vi "Resize Front Panel Main.vi"(0 "Left Listbox":refnum<vi>, 1 "Top Level VI":refnum<vi>, 2 "Stop":refnum<vi>, 3 "Number of Columns":i32=4, 7 "Left Splitter":refnum<vi>, 11 "error in (no error)":errorcluster, 12 "Left Pane Items":refnum<vi>[](array[refnum]), 13 "Mid Pane Items":refnum<vi>[](array[refnum])) -> (15 "error out":errorcluster)   [LabVIEW 2020]
uses:
  <vilib>/Utility/miscctls.llb/LVRectTypeDef.ctl
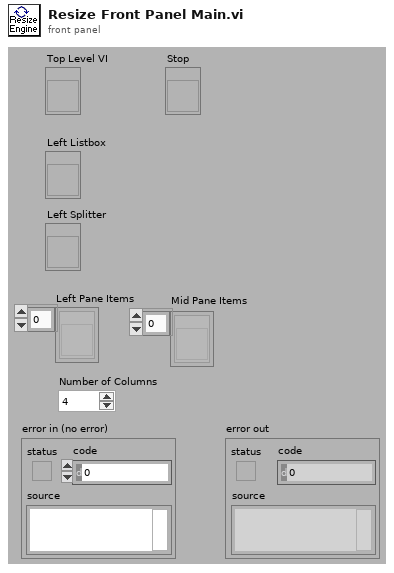
[diagram p1: front panel]
types:
  T1 = typedef "LVRectTypeDef.ctl" = cluster{"Left":i16, "Top":i16, "Right":i16, "Bottom":i16}
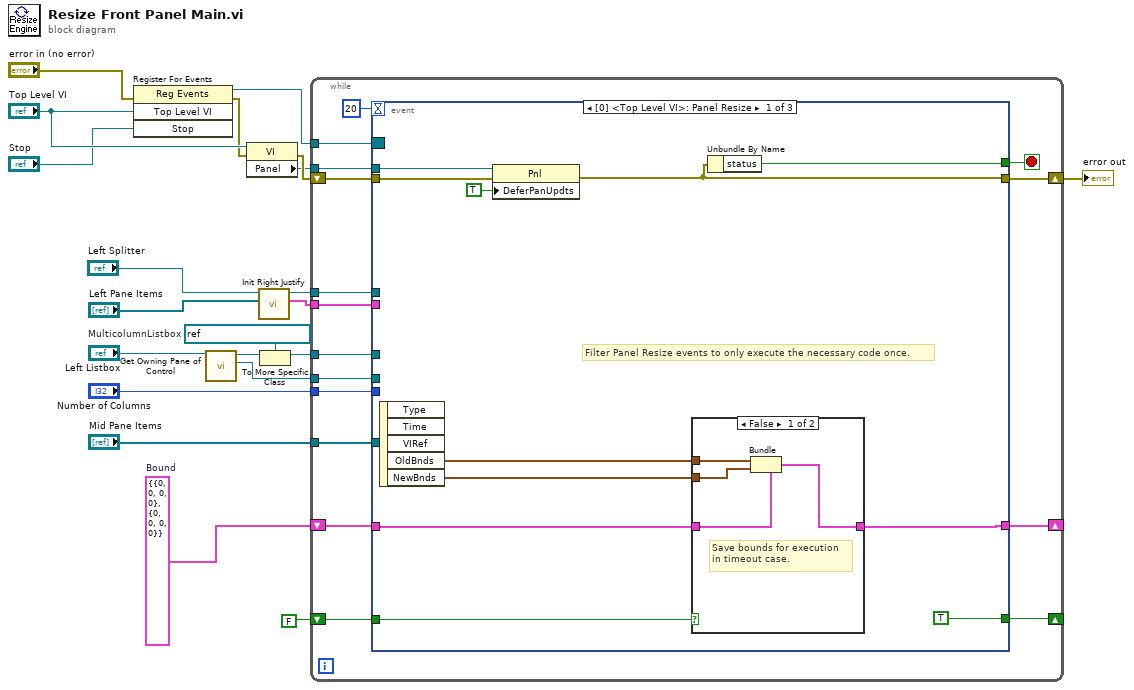
[diagram p0: block diagram]
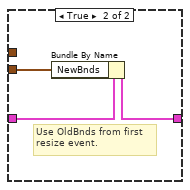
[diagram p2: hidden frame]
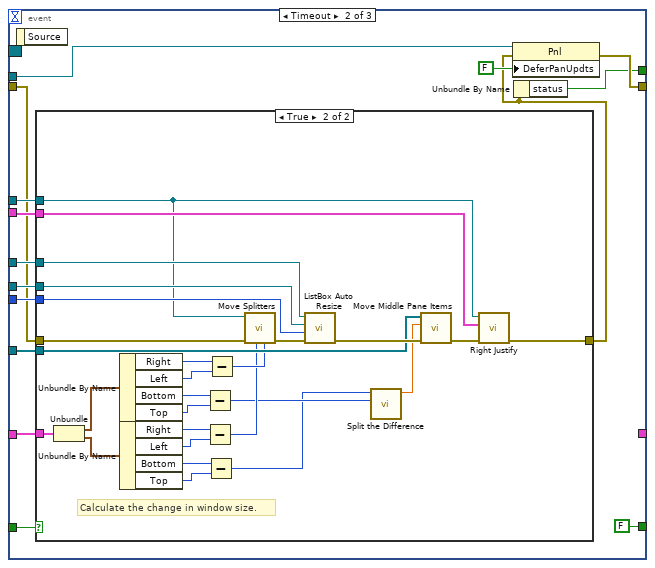
[diagram p3: hidden frame]
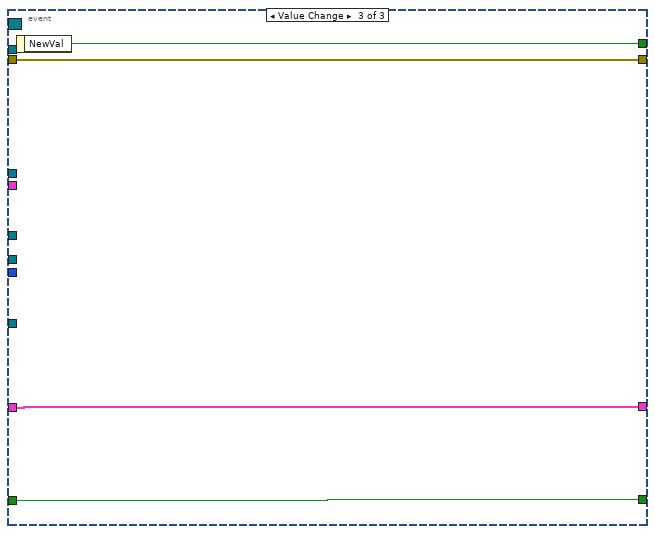
[diagram p5: hidden frame]
diagram:
  w2 = cluster{"OldBnds":T1, "NewBnds":T1} {"OldBnds"={"Left"=0, "Top"=0, "Right"=0, "Bottom"=0}, "NewBnds"={"Left"=0, "Top"=0, "Right"=0, "Bottom"=0}}  # Bound
  w4 = refnum<vi> refnum  # MulticolumnListbox
  n1 = register-events(error in="error in (no error)", "Top Level VI", "Stop") -> (reference out=w15:refnum<event-registration>, error out=w14:errorcluster)  [unwired: 1 in]
  n2 = call "Get Owning Pane of Control.vi"("Ctl Refnum"="Left Listbox") -> ("Owning Pane"=w7:refnum<vi>, "dup Ctl Refnum"=w6:refnum<vi>)  [unwired: 8 in, 1 out]
  n3 = property class="VI"(reference="Top Level VI", error in=w14) -> (error out=w13:errorcluster, "Panel"=w3:refnum<vi>)  [unwired: 1 out]
  n4 = call "Init Right Justify.vi"("Right Justified Items"="Left Pane Items", "Splitter Reference"="Left Splitter") -> ("Position Coordinates"=w18:cluster{refnum<vi>, i32}[], "Splitter Reference"=w20:refnum<vi>)  [unwired: 7 in, 1 out]
  n5 = To More Specific Class(target class=w4, reference=w6) -> (specific class reference=w5:refnum<vi>)  [unwired: 1 in, 1 out]
  n6 = while {
    tunnel: w3 -> [w36]
    tunnel: w18 -> [w34]
    tunnel: w20 -> [w33]
    tunnel: w15 -> [w32]
    tunnel: w5 -> [w31]
    shift-right: [w29] -> w9
    shift-left: w13 -> [w30]
    tunnel: "Number of Columns" -> [w28]
    tunnel: "Mid Pane Items" -> [w27]
    tunnel: w7 -> [w26]
    shift-right: [w25] -> _
    shift-left: w2 -> [w24]
    shift-right: [w23] -> _
    shift-left: FALSE -> [w22]
    stop <- w37 stop-if-true
    n7 = event shown="[0] <Top Level VI>: Panel Resize" {
      selector: w32 -> [_ _ _]
      dyn-events: _ -> [_ _ _]
      timeout: 20 -> [_ _ _]
      tunnel: [w44 w56 w102] -> w37
      tunnel: w36 -> [w48 w58 _]
      tunnel: w34 -> [_ w70 _]
      tunnel: w33 -> [_ w68 _]
      tunnel: w31 -> [_ w69 _]
      tunnel: w30 -> [w46 w60 w101]
      tunnel: [w45 w59 w101] -> w29
      tunnel: w28 -> [_ w66 _]
      tunnel: w27 -> [_ w67 _]
      tunnel: w26 -> [_ w65 _]
      tunnel: [w38 _ w100] -> w25
      tunnel: w24 -> [w39 w64 w100]
      tunnel: [TRUE FALSE w99] -> w23
      tunnel: w22 -> [w42 w62 w99]
      event Panel Resize {
        # "Filter Panel Resize events to only execute the necessary code once."
        n8 = event-data() -> ("OldBnds"=w41:T1, "NewBnds"=w40:T1)  [unwired: 1 in, 3 out]
        n9 = property class="Pnl"(reference=w48, error in=w46, "DeferPanUpdts"=TRUE ("Defer Panel Updates")) -> (error out=w45:errorcluster)  [unwired: 1 out]
        n10 = case shown="False" w42 {
          tunnel: w41 -> [w52 _]
          tunnel: w40 -> [w51 w53]
          tunnel: w39 -> [w50 w55]
          tunnel: [w49 w54] -> w38
          frame False {
            # "Save bounds for execution\nin timeout case."
            n11 = Bundle(cluster=w50, "OldBnds"=w52, "NewBnds"=w51) -> (w49:cluster{"OldBnds":T1, "NewBnds":T1})
          }
          frame True {
            # "Use OldBnds from first\nresize event."
            n12 = Bundle By Name(cluster=w55, "NewBnds"=w53) -> (w54:cluster{"OldBnds":T1, "NewBnds":T1})
          }
        }
        n13 = Unbundle By Name(w45) -> ("status"=w44:bool)
      }
      event Timeout {
        n14 = event-data() -> ()  [unwired: 1 in, 1 out]
        n15 = case shown="True" w62 {
          tunnel: w70 -> [_ w95]
          tunnel: w69 -> [_ w94]
          tunnel: w68 -> [_ w72]
          tunnel: w67 -> [_ w93]
          tunnel: w66 -> [_ w92]
          tunnel: w65 -> [_ w91]
          tunnel: [w71 w89] -> w57
          tunnel: w60 -> [w71 w88]
          tunnel: w64 -> [_ w75]
          frame False {
          }
          frame True {
            # "Calculate the change in window size."
            n16 = Unbundle(w75) -> ("OldBnds"=w74:T1, "NewBnds"=w73:T1)
            n17 = Unbundle By Name(w74) -> ("Right"=w86:i16, "Left"=w87:i16, "Bottom"=w81:i16, "Top"=w80:i16)
            n18 = Unbundle By Name(w73) -> ("Right"=w84:i16, "Left"=w83:i16, "Bottom"=w78:i16, "Top"=w77:i16)
            n19 = Subtract(x=w81, y=w80) -> (x-y=w79:i16)
            n20 = Subtract(x=w84, y=w83) -> (x-y=w82:i16)
            n21 = Subtract(x=w78, y=w77) -> (x-y=w76:i16)
            n22 = Subtract(x=w86, y=w87) -> (x-y=w85:i16)
            n23 = call "Move Splitters.vi"("Old Width"=w85, "New Width"=w82, "error in"=w88, "Left Splitter"=w72) -> ("error out"=w97:errorcluster)  [unwired: 7 in]
            n24 = call "ListBox Auto Resize.vi"("error in (no error)"=w97, "Number of Columns"=w92, "Owning Pane"=w91, "MultiColumn Listbox"=w94) -> ("error out"=w98:errorcluster)  [unwired: 7 in]
            n25 = call "Split the Difference.vi"("Y"=w79, "X"=w76) -> ("Half the Difference"=w96:dbl)  [unwired: 9 in]
            n26 = call "Move Middle Pane Items.vi"("error in"=w98, "Vertical Distance to Move"=w96, "Object References"=w93) -> ("error out"=w90:errorcluster)  [unwired: 8 in]
            n27 = call "Right Justify.vi"("error in"=w90, "Position Coordinates"=w95, "Splitter Reference"=w72) -> ("error out"=w89:errorcluster)  [unwired: 8 in]
          }
        }
        n28 = property class="Pnl"(reference=w58, error in=w57, "DeferPanUpdts"=FALSE ("Defer Panel Updates")) -> (error out=w59:errorcluster)  [unwired: 1 out]
        n29 = Unbundle By Name(w57) -> ("status"=w56:bool)
      }
      event Value Change {
        n30 = event-data() -> ("NewVal"=w102:bool)  [unwired: 1 in]
      }
    }
  }
  "error out" <- w9
